vi "Panel.Disable.vi"(8 "error in (no error)":errorcluster, 11 "Defer Panel Updates (F)":bool) -> (0 "error out":errorcluster)   [LabVIEW 2014]
panel:
  out "VI Name":string
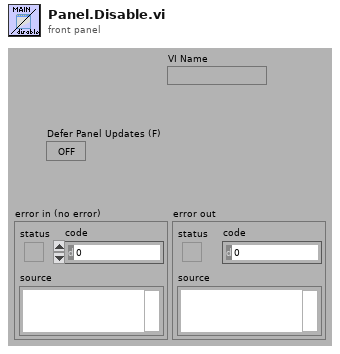
[diagram p1: front panel]
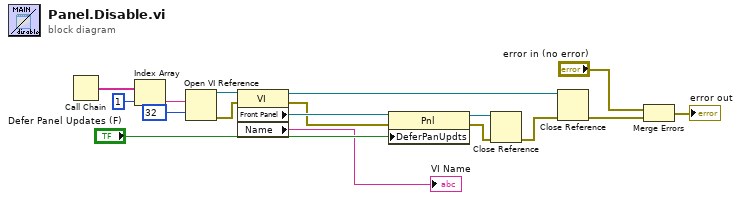
[diagram p0: block diagram]
diagram:
  n1 = Call Chain() -> (call chain=w5:string[])
  n2 = Index Array(array=w5, index=1) -> (element=w3:string)
  n3 = Open VI Reference(vi path=w3, options=32) -> (vi reference=w15:refnum<vi>, error out=w16:errorcluster)  [unwired: 2 in, 2 out]
  n4 = property class="VI"(reference=w15, error in=w16) -> (reference out=w14:refnum<vi>, error out=w10:errorcluster, "Front Panel"=w13:refnum<vi>, "Name"=→"VI Name":string)
  n5 = property class="Pnl"(reference=w13, error in=w10, "DeferPanUpdts"="Defer Panel Updates (F)") -> (reference out=w11:refnum<vi>, error out=w12:errorcluster)
  n6 = Close Reference(reference=w11, error in (no error)=w12) -> (error out=w9:errorcluster)
  n7 = Close Reference(reference=w14, error in (no error)=w9) -> (error out=w8:errorcluster)
  n8 = Merge Errors("error in (no error)", w8) -> (→"error out":errorcluster)
